vi "Adaptive Base Time.vi"(8 "Error In":errorcluster, 11 "ICT _Data":T1) -> (0 "Error Out":errorcluster, 1 "New Base Cycle Time_Out":dbl, 2 "Total Cycle Time in Seconds":dbl, 3 "SSD":string)   [LabVIEW 2016]
panel:
  out "Report Text":string
  out "Pass/Fail?":bool
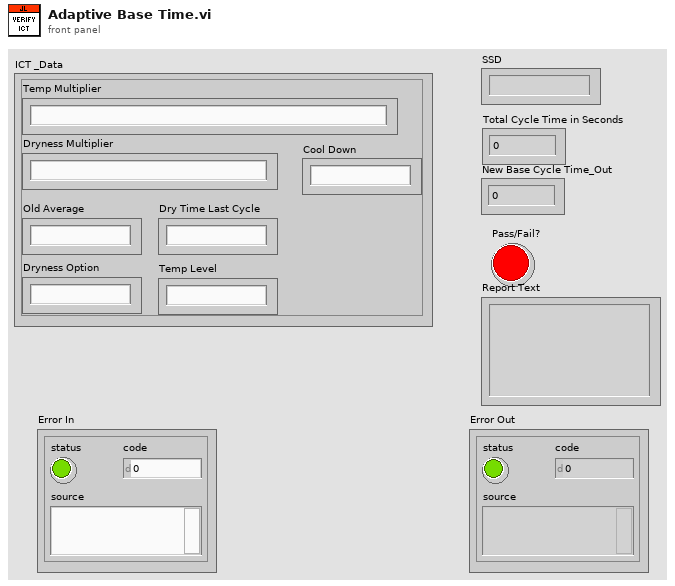
[diagram p1: front panel]
types:
  T1 = cluster{"Old Average":string, "Dry Time Last Cycle":string, "Dryness Option":string, "Temp Level":string, "Temp Multiplier":string, "Dryness Multiplier":string, "Cool Down":string}
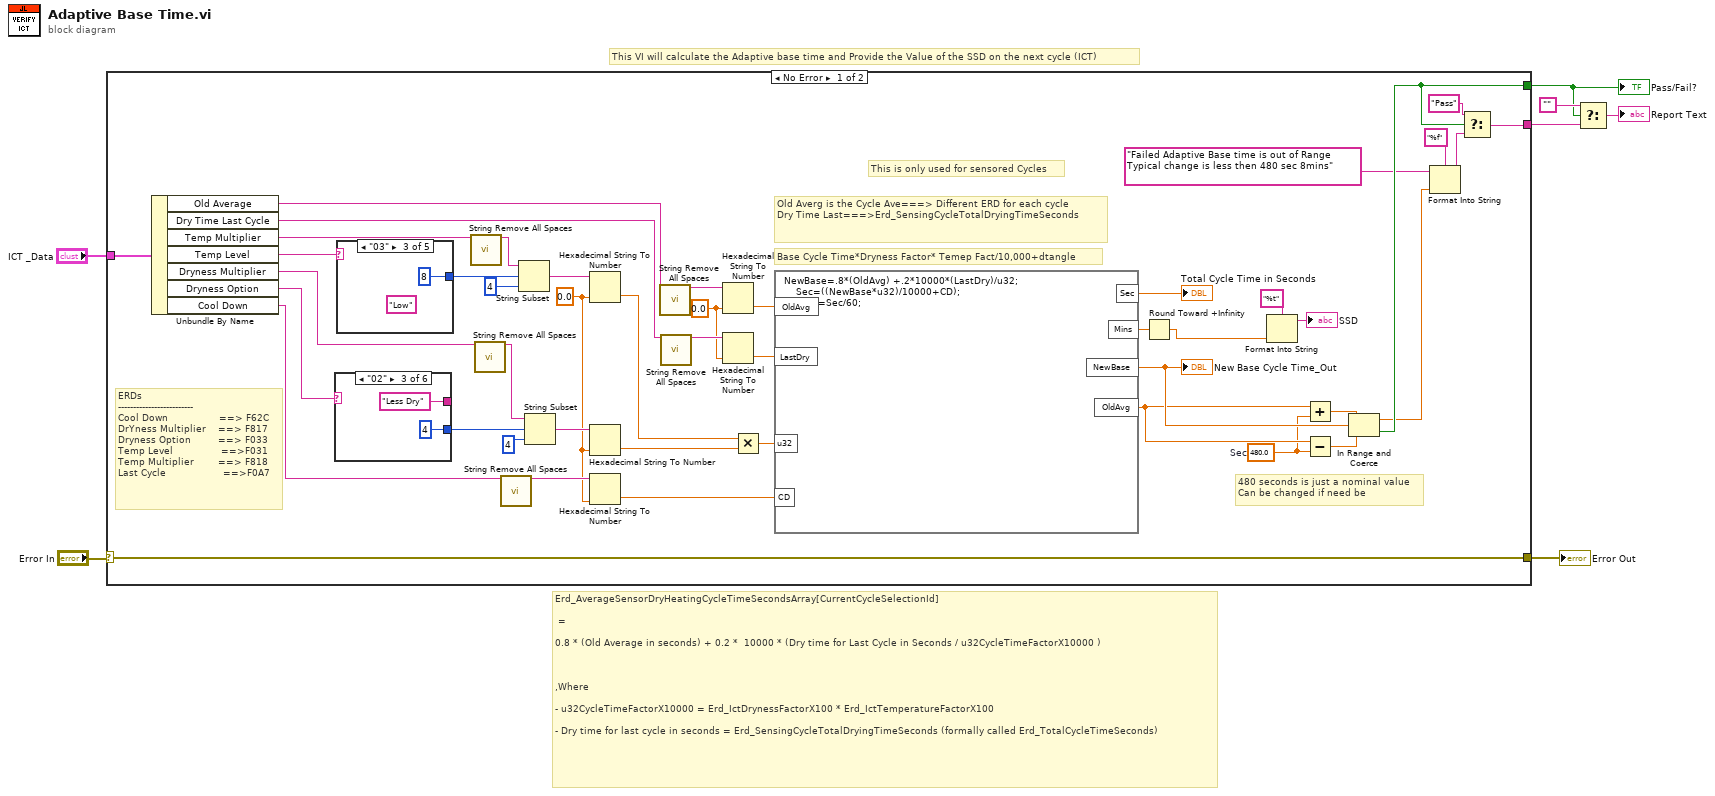
[diagram p0: block diagram]
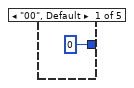
[diagram p2: hidden frame]
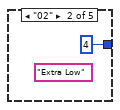
[diagram p3: hidden frame]
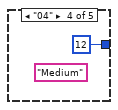
[diagram p4: hidden frame]
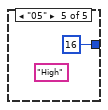
[diagram p5: hidden frame]
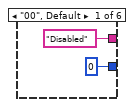
[diagram p6: hidden frame]
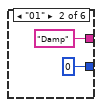
[diagram p7: hidden frame]
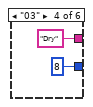
[diagram p8: hidden frame]
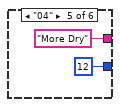
[diagram p9: hidden frame]
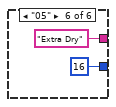
[diagram p10: hidden frame]
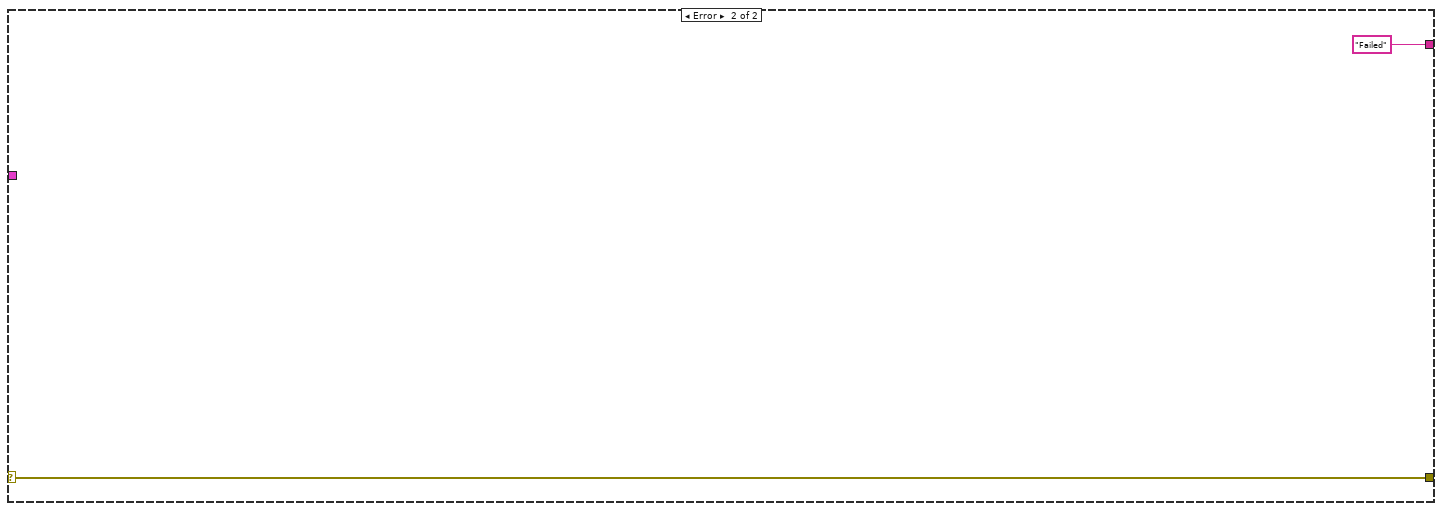
[diagram p11: hidden frame]
diagram:
  # "This VI will calculate the Adaptive base time and Provide the Value of the SSD on the next cycle (ICT)"
  # "Erd_AverageSensorDryHeatingCycleTimeSecondsArray[CurrentCycleSelectionId]\n\n =\n\n0.8 * (Old Average in seconds) + 0.2 *  10000 * (Dry time for Last Cycle in Seconds / u32CycleTimeFactorX10000 )\n\n \n\n,Where \n\n- u32CycleTimeFactorX10000 = Erd_IctDrynessFactorX100 * Erd_IctTemperatureFactorX100 \n\n- Dry time for last cycle in seconds = Erd_SensingCycleTotalDryingTimeSeconds (formally called Erd_TotalCycleTimeSeconds)"
  n1 = case shown="No Error" "Error In" {
    selector: "Error In" -> [w29 w71]
    tunnel: [w29 w71] -> w6
    tunnel: "ICT _Data" -> [w28 _]
    tunnel: [w19 _] -> w2
    tunnel: [w20 "Failed" ("f")] -> w1
    frame No Error {
      w22 = 480.0  # Sec
      w11 = 0.0
      w50 = 0.0
      # "480 seconds is just a nominal value\nCan be changed if need be"
      # "ERDs\n-------------------------\nCool Down                 ==> F62C\nDrYness Multiplier    ==> F817\nDryness Option         ==> F033\nTemp Level                ==>F031 \nTemp Multiplier        ==> F818\nLast Cycle                   ==>F0A7"
      # "This is only used for sensored Cycles"
      # "Old Averg is the Cycle Ave===> Different ERD for each cycle\nDry Time Last===>Erd_SensingCycleTotalDryingTimeSeconds"
      # "Base Cycle Time*Dryness Factor* Temep Fact/10,000+dtangle"
      n2 = Unbundle By Name(w28) -> ("Old Average"=w31:string, "Dry Time Last Cycle"=w30:string, "Temp Multiplier"=w32:string, "Temp Level"=w35:string, "Dryness Multiplier"=w33:string, "Dryness Option"=w34:string, "Cool Down"=w14:string)
      n3 = case shown="\"02\"" w34 {
        tunnel: ["Disabled" "Damp" "Less Dry" "Dry" "More Dry" "Extra Dry"] -> _
        tunnel: [0 ("offset (0)") 0 ("offset (0)") 4 ("offset (0)") 8 ("offset (0)") 12 ("offset (0)") 16 ("offset (0)")] -> w44
        frame "00", Default {
        }
        frame "01" {
        }
        frame "02" {
        }
        frame "03" {
        }
        frame "04" {
        }
        frame "05" {
        }
      }
      n4 = case shown="\"03\"" w35 {
        tunnel: [0 ("offset (0)") 4 ("offset (0)") 8 ("offset (0)") 12 ("offset (0)") 16 ("offset (0)")] -> w46
        frame "00", Default {
        }
        frame "02" {
          (unwired) "Extra Low"
        }
        frame "03" {
          (unwired) "Low"
        }
        frame "04" {
          (unwired) "Medium"
        }
        frame "05" {
          (unwired) "High"
        }
      }
      n5 = call "String Remove All Spaces.vi"("Input String"=w32) -> ("Spaces Removed"=w47:string)  [unwired: 13 in, 1 out]
      n6 = call "String Remove All Spaces.vi"("Input String"=w33) -> ("Spaces Removed"=w45:string)  [unwired: 13 in, 1 out]
      n7 = call "String Remove All Spaces.vi"("Input String"=w14) -> ("Spaces Removed"=w13:string)  [unwired: 13 in, 1 out]
      n8 = String Subset(string=w47, offset (0)=w46, length (rest)=4 ("length (rest)")) -> (substring=w42:string)
      n9 = String Subset(string=w45, offset (0)=w44, length (rest)=4 ("length (rest)")) -> (substring=w41:string)
      n10 = Hexadecimal String To Number(string=w42, default (0uL)=w11) -> (number=w40:dbl)  [unwired: 1 in, 1 out]
      n11 = Hexadecimal String To Number(string=w41, default (0uL)=w11) -> (number=w39:dbl)  [unwired: 1 in, 1 out]
      n12 = Hexadecimal String To Number(string=w13, default (0uL)=w11) -> (number=w12:dbl)  [unwired: 1 in, 1 out]
      n13 = call "String Remove All Spaces.vi"("Input String"=w31) -> ("Spaces Removed"=w51:string)  [unwired: 13 in, 1 out]
      n14 = call "String Remove All Spaces.vi"("Input String"=w30) -> ("Spaces Removed"=w52:string)  [unwired: 13 in, 1 out]
      n15 = Hexadecimal String To Number(string=w51, default (0uL)=w50) -> (number=w48:dbl)  [unwired: 1 in, 1 out]
      n16 = Hexadecimal String To Number(string=w52, default (0uL)=w50) -> (number=w49:dbl)  [unwired: 1 in, 1 out]
      n17 = Multiply(x=w40, y=w39) -> (x*y=w38:dbl)
      n18 = formula code="NewBase=.8*(OldAvg) +.2*10000*(LastDry)/u32;\n    Sec=((NewBase*u32)/10000+CD);\n    Mins=Sec/60;"("OldAvg"=w48, "LastDry"=w49, "u32"=w38, "CD"=w12) -> ("NewBase"=w26:dbl, "Mins"=w37:dbl, "Sec"=→"Total Cycle Time in Seconds":dbl, "OldAvg"=w23:dbl)
      "New Base Cycle Time_Out" <- w26
      n19 = Round Toward +Infinity(x=w37) -> (ceil(x): smallest int >= x=w10:dbl)
      n20 = Format Into String(format string="%t", w10) -> (resulting string=→"SSD":string)  [unwired: 2 in, 1 out]
      n21 = Add(x=w23, y=w22) -> (x+y=w25:dbl)
      n22 = Subtract(x=w23, y=w22) -> (x-y=w24:dbl)
      n23 = In Range and Coerce(upper limit=w25, x=w26, lower limit=w24) -> (coerced(x)=w18:dbl, In Range?=w19:bool)
      n24 = Format Into String(format string="%f", initial string="Failed Adaptive Base time is out of Range Typical change is less then 480 sec 8mins" ("string"), w18) -> (resulting string=w17:string)  [unwired: 1 in, 1 out]
      n25 = Select(t="Pass" ("f"), s=w19, f=w17) -> (s? t:f=w20:string)
    }
    frame Error {
    }
  }
  "Error Out" <- w6
  "Pass/Fail?" <- w2
  n26 = Select(t="", s=w2, f=w1) -> (s? t:f=→"Report Text":string)
